vi "pov to bool(Trigger).vi"(11 "Numeric":i16) -> (0 "Left":bool, 1 "Down":bool, 2 "Up":bool, 3 "Right":bool)   [LabVIEW 2019, in "Joysticks.lvlib" / "Joysticks.lvclass"]
doc: "This VI takes the D-Pad actions into 4 seperate outputs."
uses:
  Joysticks.lvclass
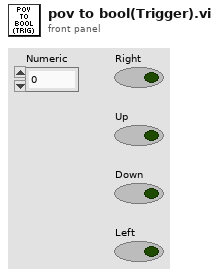
[diagram p1: front panel]
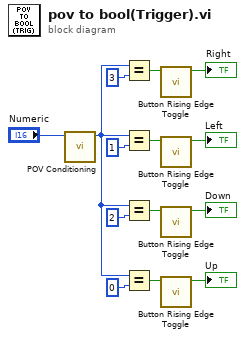
[diagram p0: block diagram]
diagram:
  n1 = call "POV Conditioning.vi"("POV"="Numeric") -> ("Output [-1-4]"=w13:i16)  [unwired: 10 in]
  n2 = Equal?(x=w13, y=i16 3) -> (x = y?=w6:bool)
  n3 = Equal?(x=w13, y=i16 1) -> (x = y?=w11:bool)
  n4 = Equal?(x=w13, y=i16 2) -> (x = y?=w5:bool)
  n5 = Equal?(x=w13, y=i16 0) -> (x = y?=w4:bool)
  n6 = call "Button Rising Edge Toggle.vi"("Button"=w6) -> ("Rising edge?"=→"Right":bool)  [unwired: 10 in]
  n7 = call "Button Rising Edge Toggle.vi"("Button"=w11) -> ("Rising edge?"=→"Left":bool)  [unwired: 10 in]
  n8 = call "Button Rising Edge Toggle.vi"("Button"=w5) -> ("Rising edge?"=→"Down":bool)  [unwired: 10 in]
  n9 = call "Button Rising Edge Toggle.vi"("Button"=w4) -> ("Rising edge?"=→"Up":bool)  [unwired: 10 in]
